vi "test4-ProcessAsyncMessageWithoutReplyInCSMLoop(SendAndReceive).vi"(8 "error in (no error)":errorcluster, 11 "TestCase in":refnum<class "testcase-CSMAddonLoopSupport.lvclass">) -> (0 "error out":errorcluster, 3 "TestCase out":refnum<class "testcase-CSMAddonLoopSupport.lvclass">)   [LabVIEW 2017, in "testcase-CSMAddonLoopSupport.lvclass"]
uses:
  testcase-CSMAddonLoopSupport.lvclass
  4585ddd5-ba69-4fd4-94fe-207595864cbd.vi
  a7620e19-6451-46a1-85ca-ade5edb58587.vi
  55fec5d7-cd22-46f7-b641-2c7c49619fc8.vi
  9cfd6824-310a-46c9-9b98-3854de5c7aa2.vi
  <vilib>/addons/_JKI Toolkits/VI Tester/TestCase.llb/TestCase.lvclass
  src/user.lib/_NEVSTOP/Communicable State Machine(CSM)/Communicable State Machine.lvlib
  C:/Program Files (x86)/National Instruments/LabVIEW 2017/vi.lib/addons/_JKI Toolkits/VI Tester/TestCase.llb/TestCase.lvclass
panel:
  out "LoopCount":i32
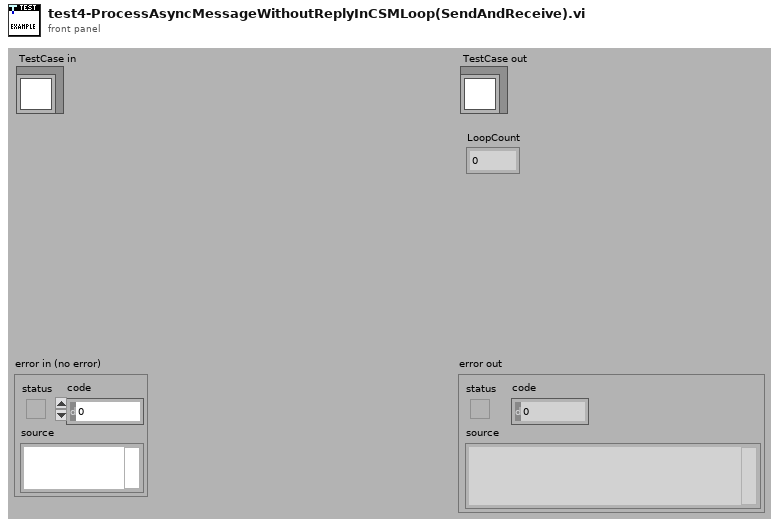
[diagram p1: front panel]
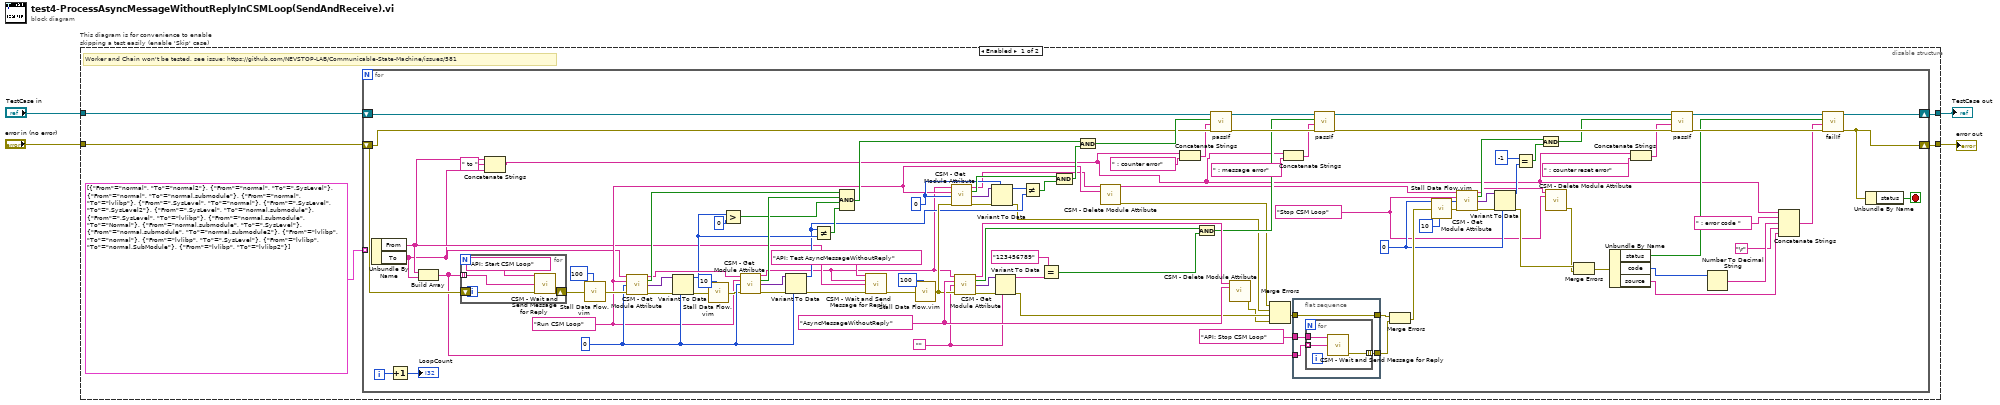
[diagram p0: block diagram]
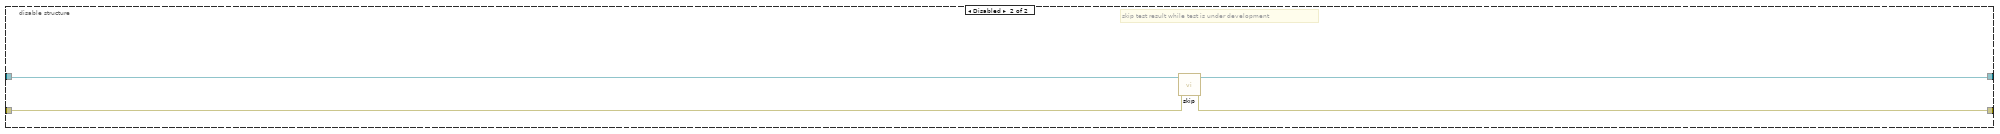
[diagram p2: hidden frame]
diagram:
  n1 = disable-structure "This diagram is for convenience to enable skipping a test easily (enable 'Skip' case)" shown="Enabled" {
    disable-tunnel: "TestCase in" -> [w9 w127]
    disable-tunnel: [w7 w125] -> w1
    disable-tunnel: [w6 w126] -> w3
    disable-tunnel: "error in (no error)" -> [w8 w124]
    frame Enabled {
      # "Worker and Chain won't be tested, see issue: https://github.com/NEVSTOP-LAB/Communicable-State-Machine/issues/581"
      n2 = for {
        tunnel: cluster{"From":string, "To":string}[] [{"From"="normal", "To"="normal2"}, {"From"="normal", "To"=".SysLevel"}, {"From"="normal", "To"="normal.submodule"}, {"From"="normal", "To"="lvlibp"}, {"From"=".SysLevel", "To"="normal"}, {"From"=".SysLevel", "To"=".SysLevel2"}, {"From"=".SysLevel", "To"="normal.submodule"}, {"From"=".SysLevel", "To"="lvlibp"}, {"From"="normal.submodule", "To"="Normal"}, {"From"="normal.submodule", "To"=".SysLevel"}, {"From"="normal.submodule", "To"="normal.submodule2"}, {"From"="lvlibp", "To"="normal"}, {"From"="lvlibp", "To"=".SysLevel"}, {"From"="lvlibp", "To"="normal.SubModule"}, {"From"="lvlibp", "To"="lvlibp2"}] -> [w33] mode=indexing
        shift-right: [w63] -> w7
        shift-left: w9 -> [w73]
        shift-right: [w62] -> w6
        shift-left: w8 -> [w64]
        i -> [w112]
        stop <- w67 stop-if-true
        w14 = ""
        w37 = "Stop CSM Loop" ("State")
        w50 = 0
        w76 = 0
        w90 = 0
        w41 = "Run CSM Loop" ("State")
        w101 = "AsyncMessageWithoutReply" ("State")
        n3 = Unbundle By Name(w33) -> ("From"=w31:string, "To"=w30:string)
        n4 = Increment(x=w112) -> (x+1=→"LoopCount":i32)
        n5 = Build Array(w31, w30) -> (w32:string[])
        n6 = for {
          shift-right: [w115] -> w110
          shift-left: w64 -> [w114]
          tunnel: w32 -> [w113] mode=indexing
          n7 = call "CSM - Wait and Send Message for Reply.vi"("State"="API: Start CSM Loop", "Target Module"=w113, "Error In (No Error)"=w114) -> ("error out"=w115:errorcluster)  [unwired: 9 in, 3 out]
        }
        n8 = Concatenate Strings(w31, " to " ("string"), w30) -> (w17:string)
        n9 = call "Stall Data Flow.vim"("value in"=w110, "milliseconds to wait"=u32 100) -> ("value out"=w98:errorcluster)  [unwired: 1 out]
        n10 = call "CSM - Get Module Attribute.vi"("CSM Name"=w30, "Attribute"=w41, "Default Value (Empty Variant)"=w90, "Error In"=w98) -> ("CSM Name (Dup)"=w92:string, "Found"=w97:bool, "Value"=w91:variant, "error out"=w95:errorcluster)  [unwired: 7 in, 1 out]
        n11 = Variant To Data(error in=w95, type=w90, Variant=w91) -> (data=w85:i32, error out=w84:errorcluster)
        n12 = call "Stall Data Flow.vim"("value in"=w84, "milliseconds to wait"=u32 10) -> ("value out"=w83:errorcluster)  [unwired: 1 out]
        n13 = Greater?(x=w85, y=0) -> (0:w88:bool)
        n14 = call "CSM - Get Module Attribute.vi"("CSM Name"=w92, "Attribute"=w41, "Default Value (Empty Variant)"=w90, "Error In"=w83) -> ("CSM Name (Dup)"=w10:string, "Found"=w96:bool, "Value"=w87:variant, "error out"=w94:errorcluster)  [unwired: 7 in, 1 out]
        n15 = Variant To Data(error in=w94, type=w90, Variant=w87) -> (data=w74:i32, error out=w93:errorcluster)
        n16 = Not Equal?(x=w74, y=w85) -> (x != y?=w86:bool)
        n17 = Compound Arithmetic op=AND(w97, w96, w88, w86) -> (w72:bool)
        n18 = call "CSM - Wait and Send Message for Reply.vi"("State"="API: Test AsyncMessageWithoutReply", "Arguments (\"\")"=w10, "Target Module"=w31, "Error In (No Error)"=w93) -> ("error out"=w106:errorcluster)  [unwired: 8 in, 3 out]
        n19 = call "Stall Data Flow.vim"("value in"=w106, "milliseconds to wait"=u32 100) -> ("value out"=w81:errorcluster)  [unwired: 1 out]
        n20 = call "CSM - Get Module Attribute.vi"("CSM Name"=w10, "Attribute"=w41, "Default Value (Empty Variant)"=w76, "Error In"=w81) -> ("CSM Name (Dup)"=w40:string, "Found"=w78:bool, "Value"=w77:variant, "error out"=w79:errorcluster)  [unwired: 7 in, 1 out]
        n21 = call "CSM - Get Module Attribute.vi"("CSM Name"=w10, "Attribute"=w101, "Default Value (Empty Variant)"=w14, "Error In"=w81) -> ("CSM Name (Dup)"=w102:string, "Found"=w103:bool, "Value"=w104:variant, "error out"=w105:errorcluster)  [unwired: 7 in, 1 out]
        n22 = Variant To Data(error in=w79, type=w76, Variant=w77) -> (data=w75:i32, error out=w39:errorcluster)
        n23 = Variant To Data(error in=w105, type=w14, Variant=w104) -> (data=w13:string, error out=w100:errorcluster)
        n24 = Not Equal?(x=w75, y=w74) -> (x != y?=w80:bool)
        n25 = Equal?(x="123456789", y=w13) -> (x = y?=w11:bool)
        n26 = Compound Arithmetic op=AND(w78, w80) -> (w71:bool)
        n27 = And(x=w72, y=w71) -> (x .and. y?=w70:bool)
        n28 = call "CSM - Delete Module Attribute.vi"("CSM Name"=w40, "Attribute"=w41) -> ("CSM Name (Dup)"=w36:string, "error out"=w38:errorcluster)  [unwired: 10 in, 2 out]
        n29 = Concatenate Strings(w17, " : counter error" ("format string")) -> (w27:string)
        n30 = And(x=w103, y=w11) -> (x .and. y?=w66:bool)
        n31 = call-dynamic "passIf.vi"("error in (no error)"=w64, "message (\"\")"=w27, "pass"=w70, "TestCase in"=w73) -> ("error out"=w68:errorcluster, "TestCase out"=w69:refnum<class "testcase-CSMAddonLoopSupport.lvclass">)  [unwired: 6 in]
        n32 = call "CSM - Delete Module Attribute.vi"("CSM Name"=w102, "Attribute"=w101) -> ("error out"=w99:errorcluster)  [unwired: 10 in, 3 out]
        n33 = Merge Errors(w38, w39, w100, w99) -> (w42:errorcluster)
        n34 = Concatenate Strings(w17, " : message error" ("format string")) -> (w25:string)
        n35 = flat-sequence {
          tunnel: "API: Stop CSM Loop" ("State") -> [w120]
          tunnel: [w119] -> w57
          tunnel: [w118] -> w43
          tunnel: w42 -> [w118]
          tunnel: w32 -> [w117]
          frame #0 {
            n36 = for {
              tunnel: w120 -> [w123]
              tunnel: [w122] -> w119 mode=indexing
              tunnel: w117 -> [w121] mode=indexing
              n37 = call "CSM - Wait and Send Message for Reply.vi"("State"=w123, "Target Module"=w121) -> ("error out"=w122:errorcluster)  [unwired: 10 in, 3 out]
            }
          }
        }
        n38 = call-dynamic "passIf.vi"("error in (no error)"=w68, "message (\"\")"=w25, "pass"=w66, "TestCase in"=w69) -> ("error out"=w59:errorcluster, "TestCase out"=w61:refnum<class "testcase-CSMAddonLoopSupport.lvclass">)  [unwired: 6 in]
        n39 = Merge Errors(w43, w57) -> (w55:errorcluster)
        n40 = call "Stall Data Flow.vim"("value in"=w55, "milliseconds to wait"=u32 10) -> ("value out"=w54:errorcluster)  [unwired: 1 out]
        n41 = call "CSM - Get Module Attribute.vi"("CSM Name"=w36, "Attribute"=w37, "Default Value (Empty Variant)"=w50, "Error In"=w54) -> ("CSM Name (Dup)"=w35:string, "Found"=w53:bool, "Value"=w51:variant, "error out"=w52:errorcluster)  [unwired: 7 in, 1 out]
        n42 = Variant To Data(error in=w52, type=w50, Variant=w51) -> (data=w49:i32, error out=w45:errorcluster)
        n43 = Equal?(x=-1, y=w49) -> (x = y?=w46:bool)
        n44 = And(x=w53, y=w46) -> (x .and. y?=w47:bool)
        n45 = call "CSM - Delete Module Attribute.vi"("CSM Name"=w35, "Attribute"=w37) -> ("error out"=w44:errorcluster)  [unwired: 10 in, 3 out]
        n46 = Merge Errors(w45, w44) -> (w34:errorcluster)
        n47 = Unbundle By Name(w34) -> ("status"=w22:bool, "code"=w16:i32, "source"=w15:string)
        n48 = Concatenate Strings(w17, " : counter reset error" ("format string")) -> (w23:string)
        n49 = call-dynamic "passIf.vi"("error in (no error)"=w59, "message (\"\")"=w23, "pass"=w47, "TestCase in"=w61) -> ("error out"=w58:errorcluster, "TestCase out"=w60:refnum<class "testcase-CSMAddonLoopSupport.lvclass">)  [unwired: 6 in]
        n50 = Number To Decimal String(number=w16) -> (decimal integer string=w20:string)  [unwired: 1 in]
        n51 = Concatenate Strings(w17, " : error code " ("format string"), w20, "\r", w15) -> (w18:string)
        n52 = call-dynamic "failIf.vi"("error in (no error)"=w58, "message (\"\")"=w18, "fail"=w22, "TestCase in"=w60) -> ("error out"=w62:errorcluster, "TestCase out"=w63:refnum<class "testcase-CSMAddonLoopSupport.lvclass">)  [unwired: 6 in]
        n53 = Unbundle By Name(w62) -> ("status"=w67:bool)
      }
    }
    frame Disabled {
      # "skip test result while test is under development"
      n54 = call <vilib>:"skip.vi"("error in (no error)"=w124, "TestCase in"=w127) -> ("error out"=w126:errorcluster, "TestCase out"=w125:refnum<class "testcase-CSMAddonLoopSupport.lvclass">)  [unwired: 8 in]
    }
  }
  "error out" <- w3
  "TestCase out" <- w1
